vi "Impureza Superior.vi"() -> ()   [LabVIEW 2020]
panel:
  in  "?":bool
  out "Impureza \nDetectada":bool
  out "error out":errorcluster
  out "Image Out":T1(plugin-control)
  # "Teste de Impureza"
  # "Sample \nPositiva"
  # "Sample\nNegativa"
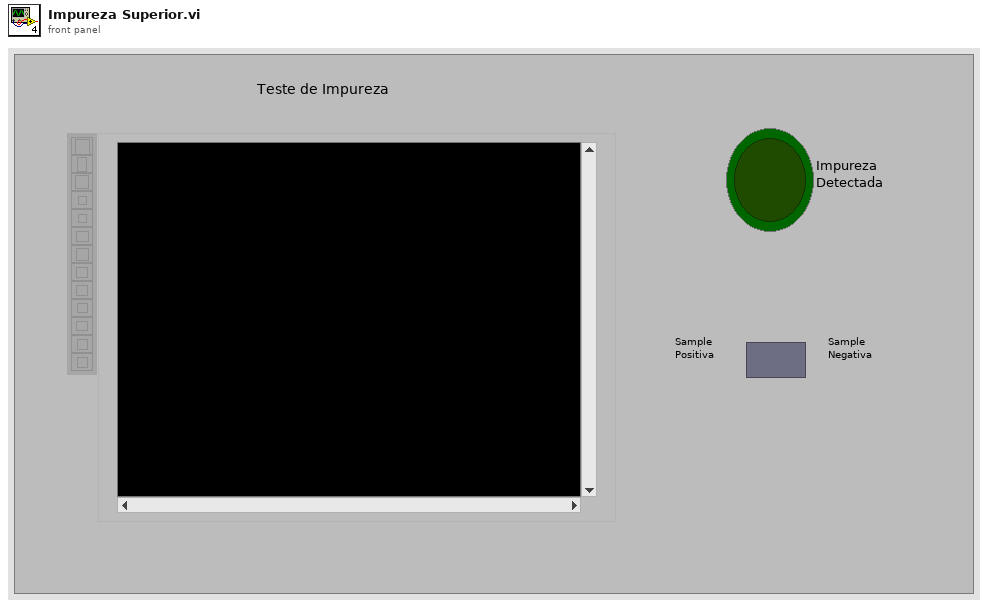
[diagram p1: front panel]
types:
  T1 = typedef "IMAQ Image.ctl" = refnum<image>
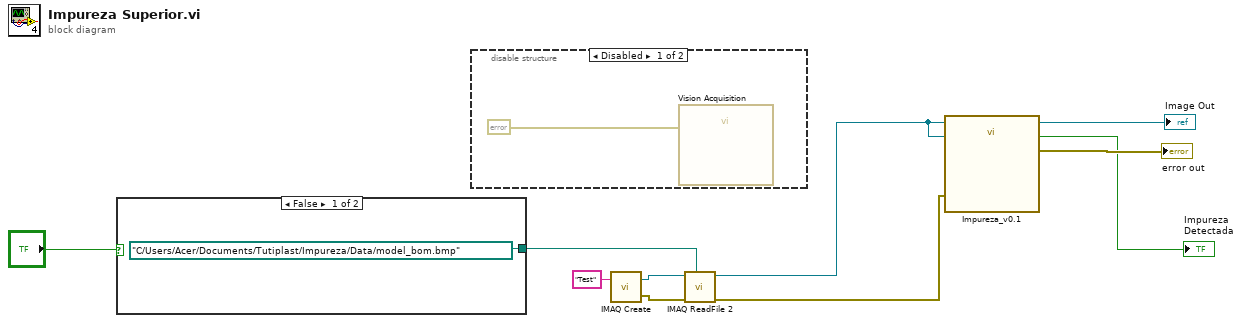
[diagram p0: block diagram]
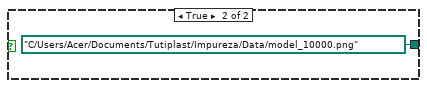
[diagram p3: hidden frame]
diagram:
  n1 = case shown="False" "?" {
    tunnel: [path "C:/Users/Acer/Documents/Tutiplast/Impureza/Data/model_bom.bmp" ("File Path") path "C:/Users/Acer/Documents/Tutiplast/Impureza/Data/model_10000.png" ("File Path")] -> w5
    frame False {
    }
    frame True {
    }
  }
  n2 = disable-structure shown="Disabled" {
    frame Disabled {
      n3 = call "Vision Acquisition"("error in"=errorcluster {"status"=FALSE, "code"=0, "source"=""}) -> ()  [unwired: 25 in, 2 out]
    }
    frame Enabled {
    }
  }
  n4 = call "IMAQ Create"("Image Name"="Test") -> ("New Image"=w6:T1, "error out"=w3:errorcluster)  [unwired: 4 in]
  n5 = call "IMAQ ReadFile 2"("File Path"=w5, "error in (no error)"=w3, "Image"=w6) -> ("error out"=w2:errorcluster, "Image Out"=w4:T1)  [unwired: 4 in, 3 out]
  n6 = call "Impureza_v0.1.vi"("Image In"=w4, "Image Dst"=w4, "error in"=w2) -> ("Image Out"=→"Image Out":T1, "Reprovado"=→"Impureza \nDetectada":bool, "error out"=→"error out":errorcluster)  [unwired: 22 in]
